vi "Field of View Microns Conversion.vi"(5 "Pixel Count":dbl, 6 "Field of View (um)":dbl) -> (1 "Microns per pixel":dbl, 2 "Field Size (5-255)":dbl)   [LabVIEW 2020]
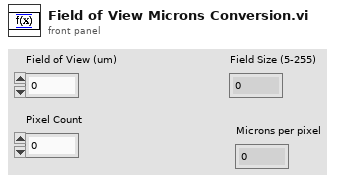
[diagram p1: front panel]
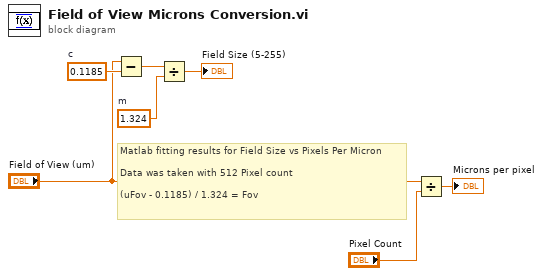
[diagram p0: block diagram]
diagram:
  w3 = 1.324  # m
  w5 = 0.1185  # c
  # "Matlab fitting results for Field Size vs Pixels Per Micron\n\nData was taken with 512 Pixel count\n\n(uFov - 0.1185) / 1.324 = Fov"
  n1 = Subtract(x="Field of View (um)", y=w5) -> (x-y=w4:dbl)
  n2 = Divide(x=w4, y=w3) -> (x/y=→"Field Size (5-255)":dbl)
  n3 = Divide(x="Field of View (um)", y="Pixel Count") -> (x/y=→"Microns per pixel":dbl)
